vi "odch_std (SubVI).vi"(11 "Gaussian noise pattern":dbl[](array[numeric])) -> (2 "odchylenie standardowe":dbl, 3 "estymator nieobciazany wariancji":dbl)   [LabVIEW 2025]
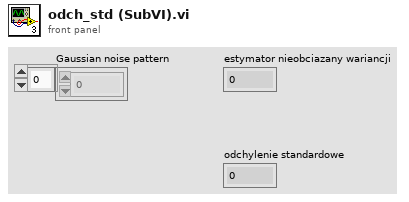
[diagram p1: front panel]
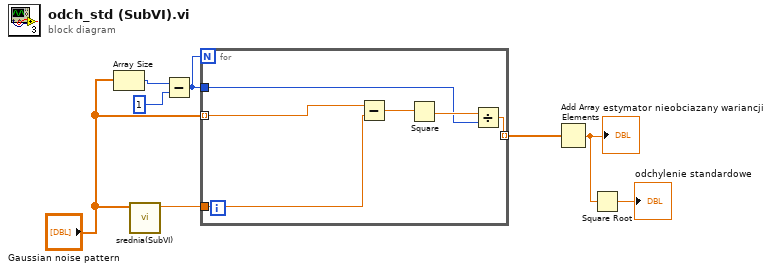
[diagram p0: block diagram]
diagram:
  n1 = Array Size(array="Gaussian noise pattern") -> (size(s)=w2:i32)
  n2 = call "srednia(SubVI).vi"("input"="Gaussian noise pattern") -> ("arytm"=w1:dbl)  [unwired: 8 in, 2 out]
  n3 = Subtract(x=w2, y=1) -> (x-y=w4:i32)
  n4 = for {
    N: w4 -> [_]
    tunnel: w1 -> [w14]
    tunnel: "Gaussian noise pattern" -> [w13] mode=indexing
    tunnel: w4 -> [w10]
    tunnel: [w9] -> w5 mode=indexing
    n5 = Subtract(x=w13, y=w14) -> (x-y=w12:dbl)
    n6 = Square(x=w12) -> (x^2=w11:dbl)
    n7 = Divide(x=w11, y=w10) -> (x/y=w9:dbl)
  }
  n8 = Add Array Elements(numeric array=w5) -> (sum=w6:dbl)
  "estymator nieobciazany wariancji" <- w6
  n9 = Square Root(x=w6) -> (sqrt(x)=→"odchylenie standardowe":dbl)
